vi "ReadCreateEnum__slk_mt.vi"(8 "error in (no error)":errorcluster, 11 "refnum in":T1) -> (0 "error out":errorcluster, 2 "create enum configure":T2, 3 "refnum out":T1)   [LabVIEW 2015, in "Lazyboots Menu Tool.lvlib"]
doc: "Gets configure datum of Create Enum.\n\n<b>[Create Enum]</b>\nControl Style = \"Classic Style\"\nNew = \"TRUE\""
uses:
  <vilib>/SLK/Lazyboots Menu Tool/Library/Lazyboots Menu Tool.lvlib
  <vilib>/SLK/Lazyboots Menu Tool/Private/CreateEnum/TypeDef/TypeDef_CreateEnumConfigure__slk_mt.ctl
  <vilib>/Utility/config.llb/Config Data RefNum.ctl
  <vilib>/Utility/config.llb/Read Key (String).vi
  <vilib>/Utility/config.llb/Read Key (Boolean).vi
  <vilib>/Utility/config.llb/NI_LVConfig.lvlib
panel:
  # "ReadCreateEnum__slk_mt.vi\nGets configure datum of Create Enum.\n\nNOTICE -- YOU MUST LEAVE THIS NOTICE IN PLACE.\n\nCopyright (c) 2011, LIANG LIU Shawn.Liu.cn@gmail.com\nAll rights reserved.\n\nRedistribution and use in source and binary forms, with or without modification, are permitted provided that the following conditions are met:\n-Redistributions of source code must retain the above copyright notice, this list of conditions and the following disclaimer.\n-Redistributions in binary form must reproduce the above copyright notice, this list of conditions and the following disclaimer in the documentation and/or other materials provided with the distribution.\n-Neither the name of the eLp nor the names of its contributors may be used to endorse or promote products derived from this software without specific prior written permission.\n\nTHIS SOFTWARE IS PROVIDED BY THE COPYRIGHT HOLDERS AND CONTRIBUTORS \"AS IS\" AND ANY EXPRESS OR IMPLIED WARRANTIES, INCLUDING, BUT NOT LIMITED TO, THE IMPLIED WARRANTIES OF MERCHANTABILITY AND FITNESS FOR A PARTICULAR PURPOSE ARE DISCLAIMED. IN NO EVENT SHALL THE COPYRIGHT HOLDER OR CONTRIBUTORS BE LIABLE FOR ANY DIRECT, INDIRECT, INCIDENTAL, SPECIAL, EXEMPLARY, OR CONSEQUENTIAL DAMAGES (INCLUDING, BUT NOT LIMITED TO, PROCUREMENT OF SUBSTITUTE GOODS OR SERVICES; LOSS OF USE, DATA, OR PROFITS; OR BUSINESS INTERRUPTION) HOWEVER CAUSED AND ON ANY THEORY OF LIABILITY, WHETHER IN CONTRACT, STRICT LIABILITY, OR TORT (INCLUDING NEGLIGENCE OR OTHERWISE) ARISING IN ANY WAY OUT OF THE USE OF THIS SOFTWARE, EVEN IF ADVISED OF THE POSSIBILITY OF SUCH DAMAGE."
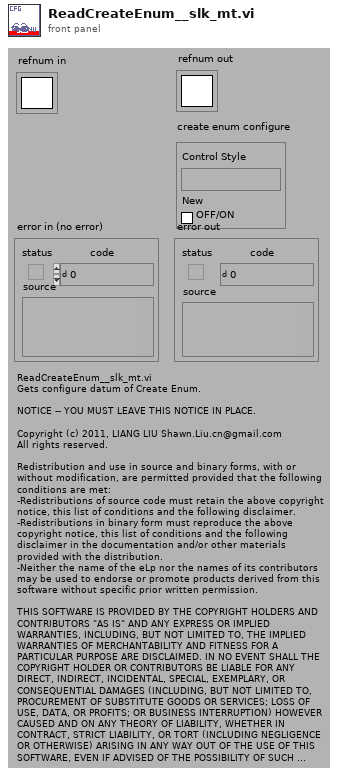
[diagram p1: front panel]
types:
  T1 = typedef "NI_LVConfig.lvlib/Config Data RefNum.ctl" = refnum<k1>
  T2 = typedef "Lazyboots Menu Tool.lvlib/TypeDef_CreateEnumConfigure__slk_mt.ctl" = cluster{"Control Style":string, "New":bool}
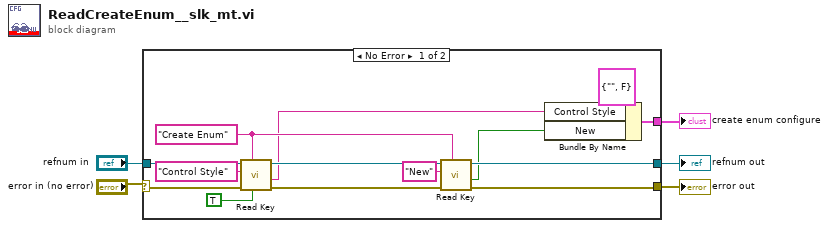
[diagram p0: block diagram]
diagram:
  n1 = case shown="No Error" "error in (no error)" {
    selector: "error in (no error)" -> [w12 w21]
    tunnel: "refnum in" -> [w17 w20]
    tunnel: [w16 w20] -> w4
    tunnel: [w11 _] -> w2
    tunnel: [w9 w21] -> w1
    frame No Error {
      w19 = "Create Enum" ("section")
      n2 = call-poly <vilib>:"Read Key.vi"("read raw string? (F)"=TRUE, "section"=w19, "error in (no error)"=w12, "key"="Control Style", "refnum"=w17) -> ("error out"=w10:errorcluster, "value"=w14:string, "refnum out"=w18:T1)  [unwired: 3 in, 1 out]
      n3 = call-poly <vilib>:"Read Key.vi"("section"=w19, "error in (no error)"=w10, "key"="New", "refnum"=w18) -> ("error out"=w9:errorcluster, "value"=w13:bool, "refnum out"=w16:T1)  [unwired: 4 in, 1 out]
      n4 = Bundle By Name(cluster=T2 {"Control Style"="", "New"=FALSE} ("Create Enum Configure"), "Control Style"=w14, "New"=w13) -> (w11:T2)
    }
    frame Error {
    }
  }
  "create enum configure" <- w2
  "error out" <- w1
  "refnum out" <- w4
